vi "Sort descending by Version.vi"(11 "Array":string[](array[string])) -> (3 "Sorted Pointers":i32[](array[numeric]))   [LabVIEW 2017, in "_Try Beta Version of CSMF.lvlib"]
uses:
  _Try Beta Version of CSMF.lvlib
  a22b5665-db45-4f9a-9afa-b29cc0b82249.vi
  284acc8e-be08-4f5a-b93f-fd922d42fb5b.vi
  a22b5665-db45-4f9a-9afa-b29cc0b82249.vi/4443fd46-6fa0-42fe-b173-791422f8c268.vi
  a22b5665-db45-4f9a-9afa-b29cc0b82249.vi/6d53486d-9fa3-4d68-a12f-868746fe63e7.vi
  a22b5665-db45-4f9a-9afa-b29cc0b82249.vi/0f454a58-6c15-4936-bc29-faa145c60f00.vi
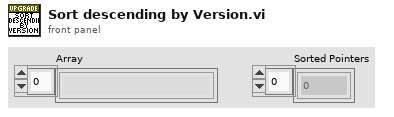
[diagram p1: front panel]
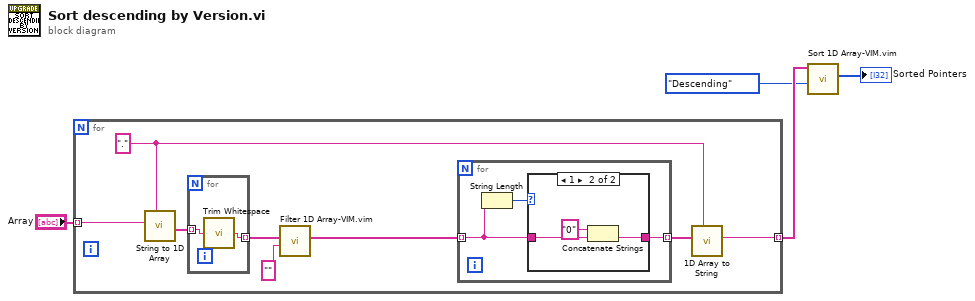
[diagram p0: block diagram]
diagram:
  n1 = for {
    tunnel: [w7] -> w3 mode=indexing
    tunnel: "Array" -> [w5] mode=indexing
    w6 = "." ("delimiter (Tab)")
    n2 = call "String to 1D Array.vi"("delimiter (Tab)"=w6, "string"=w5) -> ("Array of Strings"=w12:string[])  [unwired: 9 in]
    n3 = for {
      tunnel: w12 -> [w14] mode=indexing
      tunnel: [w13] -> w11 mode=indexing
      n4 = call <vilib>:"Trim Whitespace.vi"("string"=w14) -> ("trimmed string"=w13:string)  [unwired: 1 in]
    }
    n5 = call "Filter 1D Array-VIM.vim"("Item(s) to Filter"="" ("delimiter (Tab)"), "Array"=w11) -> ("Filtered Array"=w9:string[])  [unwired: 5 in, 1 out]
    n6 = for {
      tunnel: w9 -> [w15] mode=indexing
      tunnel: [w16] -> w8 mode=indexing
      n7 = String Length(string=w15) -> (length=w17:i32)
      n8 = case shown="1" w17 {
        tunnel: [w18 w20] -> w16
        tunnel: w15 -> [w18 w21]
        frame Default {
        }
        frame 1 {
          n9 = Concatenate Strings("0" ("string"), w21) -> (w20:string)
        }
      }
    }
    n10 = call "1D Array to String.vi"("delimiter (Tab)"=w6, "Array of Strings"=w8) -> ("delimited string"=w7:string)  [unwired: 9 in]
  }
  n11 = call "Sort 1D Array-VIM.vim"("Order (ascending)"=enum16{"Ascending", "Descending"}."Descending" ("Order (Ascending)"), "Array in"=w3) -> ("Sorted Pointers"=→"Sorted Pointers":i32[])  [unwired: 8 in, 1 out]
